vi "I2C Write.vi"(0 "Arduino Resource":T1={"COM Port"="", "Board Type"=enum."ChipKit uC32", "Connection Type"=enum."USB / Serial", "Baud Rate (115200)"=15, "Bytes Per Packet (15)"=15}, 5 "Address (0)":u8, 9 "I2C Data Bytes":u8[](array[numeric]), 11 "error in":errorcluster) -> (4 "Arduino Resource":T1={"COM Port"="", "Board Type"=enum."ChipKit uC32", "Connection Type"=enum."USB / Serial", "Baud Rate (115200)"=15, "Bytes Per Packet (15)"=15}, 15 "error out":errorcluster)   [LabVIEW 2011, in "LabVIEW Interface for ChipKit.lvlib"]
doc: "Write data to the I2C bus."
uses:
  LabVIEW Interface for ChipKit.lvlib
  Private/Type Defs/Chipkit Resource.ctl
  Private/Type Defs/Board Type.ctl
  Private/Type Defs/Connection Type.ctl
  Private/Type Defs/Command.ctl
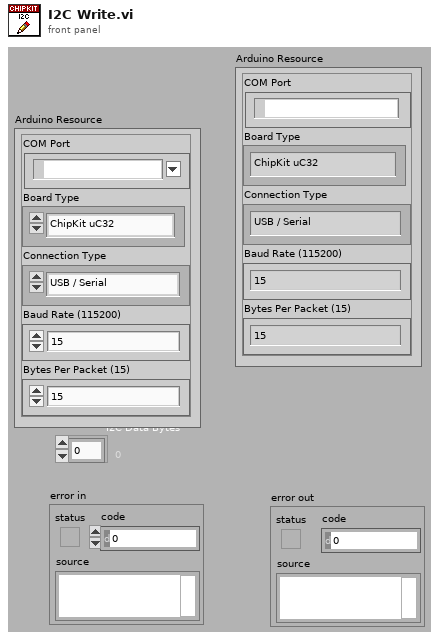
[diagram p1: front panel]
types:
  T1 = typedef "LabVIEW Interface for ChipKit.lvlib/Chipkit Resource.ctl" = cluster{"COM Port":refnum<visa-resource-name>, "Board Type":T2, "Connection Type":T3, "Baud Rate (115200)":u32, "Bytes Per Packet (15)":u32}
  T2 = typedef "LabVIEW Interface for ChipKit.lvlib/Board Type.ctl" = enum16{"ChipKit uC32", "ChipKit Uno32", "ChipKit Max32"}
  T3 = typedef "LabVIEW Interface for ChipKit.lvlib/Connection Type.ctl" = enum8{"USB / Serial", "XBEE", "BlueSmirf (Bluetooth)"}
  T4 = typedef "LabVIEW Interface for ChipKit.lvlib/Command.ctl" = enum8{"setArduinoMode", "flushSerial", "setPinMode", "digitalWritePin", "digitalWritePort", "tone", "digitalReadPin", "digitalReadPort", "analogReadPin", "analogReadPort", "pwmWritePin", "pwmWritePort", "sevenSegment_Configure", "sevenSegment_Write", "I2C Init", "I2C Write", "I2C Read", "SPI Init", "SPI Set Bit Order", "SPI Set Clock Divider", "SPI Set Data Mode", "SPI Send / Receive", "SPI Close", "Servo Set Num Servos", "Servo Config Servo", "Servo Write Angle", "Servo Read Angle", "Servo Write Pulse Width", "Servo Read Pulse Width", "Servo Detach", "LCD Init", "LCD Set Size", "LCD Set Cursor Mode", "LCD Clear", "LCD Set Cursor Position", "LCD Print", "LCD Display Power", "LCD Scroll Display", "LCD Autoscroll", "LCD Print Direction", "LCD Create Custom Char", "LCD Print Custom Char", "contAcqOn", "contAcqOff", "getFirmwareVersion", "FiniteSampleStart"}
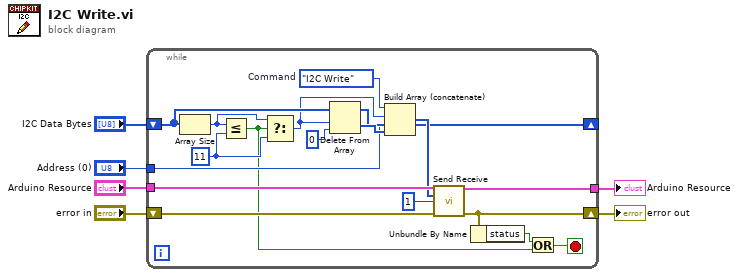
[diagram p0: block diagram]
diagram:
  n1 = while {
    tunnel: "Arduino Resource" -> [w23]
    tunnel: [w22] -> w4
    shift-right: [w18] -> _
    shift-left: "I2C Data Bytes" -> [w16]
    shift-right: [w10] -> w2
    shift-left: "error in" -> [w13]
    tunnel: "Address (0)" -> [w12]
    stop <- w8 stop-if-true
    w14 = 11 ("y")
    w24 = Command."I2C Write"  # Command
    n2 = Array Size(array=w16) -> (size(s)=w15:i32)
    n3 = Less Or Equal?(x=w15, y=w14) -> (x <= y?=w7:bool)
    n4 = Select(t=w15, s=w7, f=w14) -> (s? t:f=w11:i32)
    n5 = Delete From Array(array=w16, length=w11, index=0 ("length")) -> (deleted portion=w19:u8[], array with subset deleted=w18:u8[])
    n6 = Build Array (concatenate)(w24, w11, w12, w19) -> (w20:i32[])
    n7 = call "Send Receive.vi"("Arduino Resource"=w23, "Data"=w20, "Bytes To Read (0)"=u8 1, "error in"=w13) -> ("Arduino Resource"=w22:T1, "error out"=w10:errorcluster)  [unwired: 9 in, 1 out]
    n8 = Unbundle By Name(w10) -> ("status"=w9:bool)
    n9 = Or(x=w9, y=w7) -> (x .or. y?=w8:bool)
  }
  "error out" <- w2
  "Arduino Resource" <- w4
